vi "VelocityCommand.vi"(5 "intervalo":dbl=0.016, 7 "estimatives":T1, 8 "Velocities Y":dbl[](array[numeric]), 9 "Time Y":dbl[](array[numeric]), 10 "Velocities X":dbl[](array[numeric]), 11 "Time X":dbl[](array[numeric])) -> (1 "Vy":dbl, 2 "Vx":dbl)   [LabVIEW 2018]
panel:
  out "Velocity Profile Y":cluster{dbl[], dbl[]}[](graph)
  out "Velocity Profile X":cluster{dbl[], dbl[]}[](graph)
  in  "est_vx":dbl
  in  "est_vy":dbl
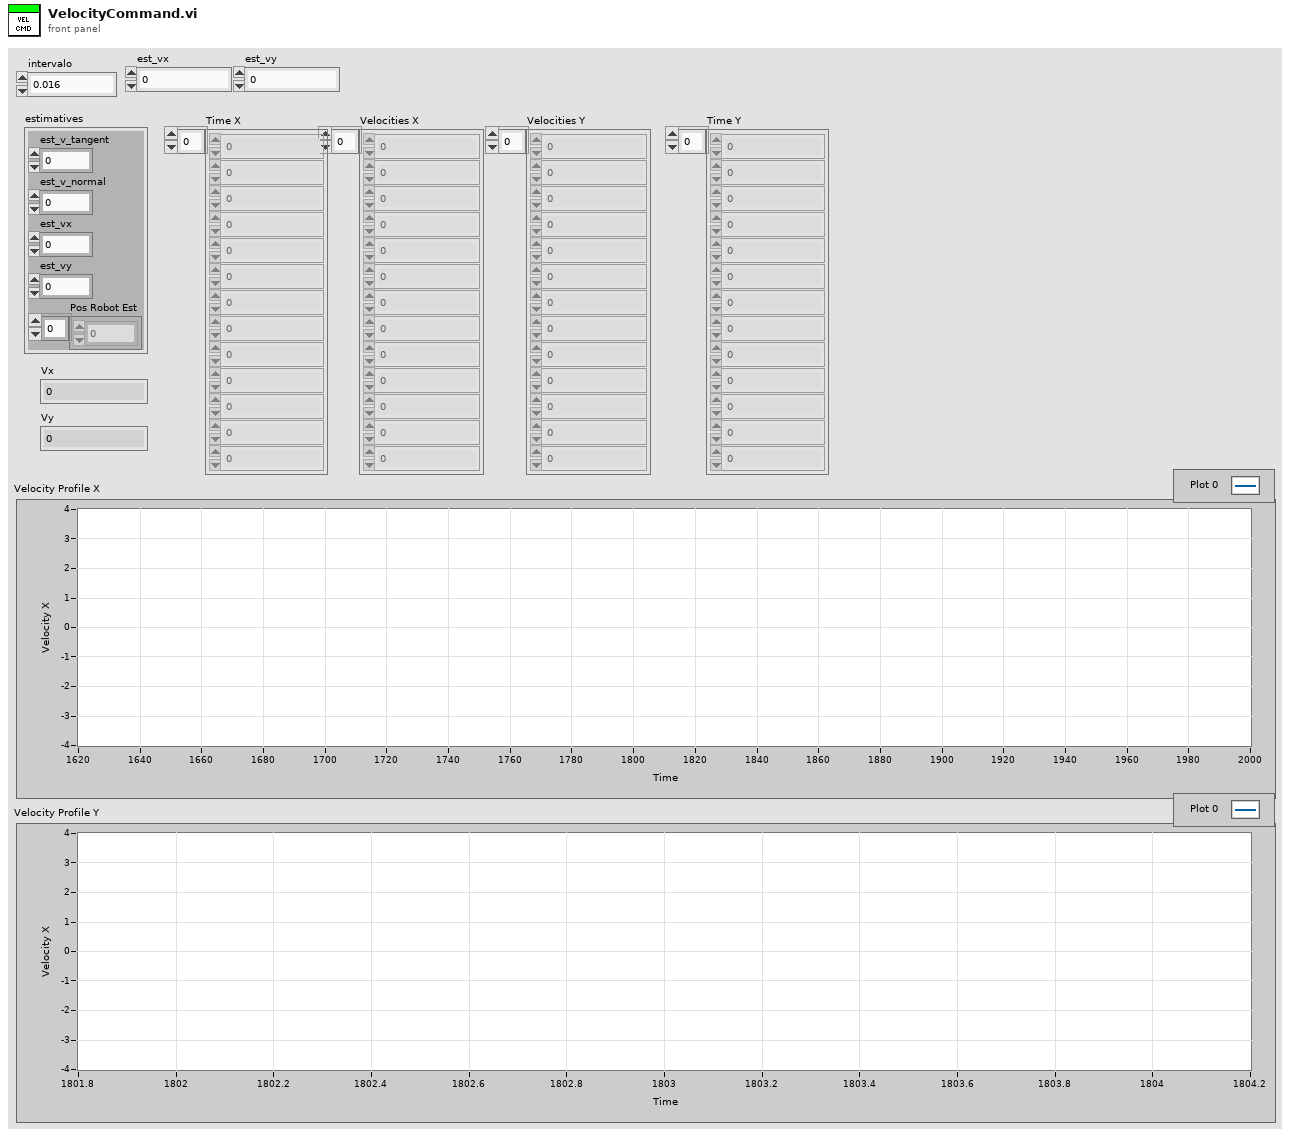
[diagram p1: front panel]
types:
  T1 = cluster{"est_v_tangent":dbl, "est_v_normal":dbl, "est_vx":dbl, "est_vy":dbl, "Pos Robot Est":dbl[]}
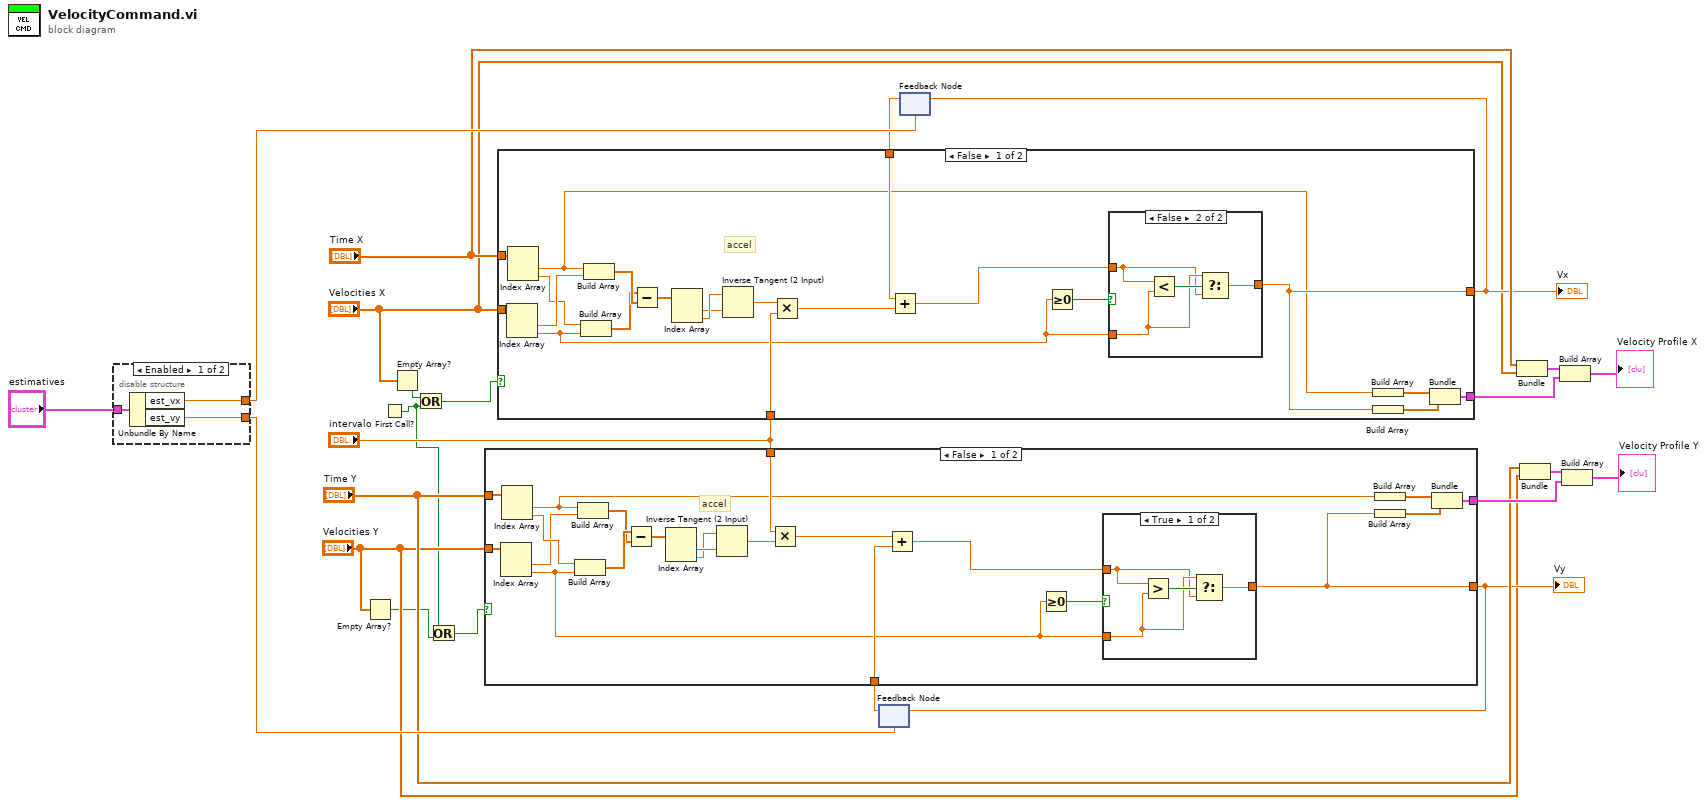
[diagram p0: block diagram]
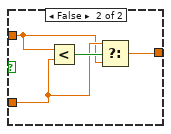
[diagram p2: hidden frame]
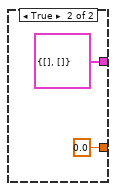
[diagram p3: hidden frame]
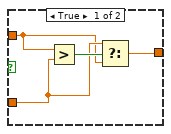
[diagram p4: hidden frame]
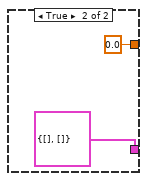
[diagram p5: hidden frame]
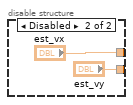
[diagram p6: hidden frame]
diagram:
  n1 = disable-structure shown="Enabled" {
    disable-tunnel: "estimatives" -> [w26 _]
    disable-tunnel: [w25 "est_vx"] -> w22
    disable-tunnel: [w24 "est_vy"] -> w20
    frame Enabled {
      n2 = Unbundle By Name(w26) -> ("est_vx"=w25:dbl, "est_vy"=w24:dbl)
    }
    frame Disabled {
    }
  }
  n3 = Empty Array?(array="Velocities Y") -> (empty?=w3:bool)
  n4 = First Call?() -> (First Call?: T/F=w2:bool)
  n5 = Empty Array?(array="Velocities X") -> (empty?=w5:bool)
  n6 = Or(x=w5, y=w2) -> (x .or. y?=w4:bool)
  n7 = Or(x=w2, y=w3) -> (x .or. y?=w1:bool)
  n8 = feedback #1(w20) -> (w8:dbl)
  n9 = case shown="False" w1 {
    tunnel: "intervalo" -> [w49 _]
    tunnel: [w48 cluster{dbl[], dbl[]} {[], []}] -> w15
    tunnel: "Velocities Y" -> [w47 _]
    tunnel: "Time Y" -> [w46 _]
    tunnel: w8 -> [w45 _]
    tunnel: [w44 0.0 ("v3")] -> w7
    frame False {
      # "accel"
      n10 = Index Array(array=w47) -> (element #1=w37:dbl, element #2=w32:dbl)  [unwired: 2 in]
      n11 = Index Array(array=w46) -> (element #1=w29:dbl, element #2=w38:dbl)  [unwired: 2 in]
      n12 = Build Array(w38, w32) -> (w40:dbl[])
      n13 = Build Array(w29, w37) -> (w39:dbl[])
      n14 = Subtract(x=w40, y=w39) -> (x-y=w41:dbl[])
      n15 = Index Array(array=w41) -> (element #1=w43:dbl, element #2=w42:dbl)  [unwired: 2 in]
      n16 = Inverse Tangent (2 Input)(1:w43, 2:w42) -> (0:w36:dbl)
      n17 = Multiply(x=w49, y=w36) -> (x*y=w35:dbl)
      n18 = Add(x=w35, y=w45) -> (x+y=w33:dbl)
      n19 = Greater Or Equal To 0?(x=w32) -> (x >= 0?=w34:bool)
      n20 = case shown="True" w34 {
        tunnel: w33 -> [w51 w55]
        tunnel: w32 -> [w52 w56]
        tunnel: [w50 w54] -> w44
        frame True {
          n21 = Greater?(x=w51, y=w52) -> (0:w53:bool)
          n22 = Select(t=w52, s=w53, f=w51) -> (s? t:f=w50:dbl)
        }
        frame False {
          n23 = Less?(x=w55, y=w56) -> (x < y?=w57:bool)
          n24 = Select(t=w56, s=w57, f=w55) -> (s? t:f=w54:dbl)
        }
      }
      n25 = Build Array(w29) -> (w31:dbl[])
      n26 = Build Array(w44) -> (w30:dbl[])
      n27 = Bundle(w31, w30) -> (w48:cluster{dbl[], dbl[]})  [unwired: 1 in]
    }
    frame True {
    }
  }
  "Vy" <- w7
  n28 = feedback-in #1(w7) -> ()
  n29 = feedback #2(w22) -> (w11:dbl)
  n30 = case shown="False" w4 {
    tunnel: "intervalo" -> [w80 _]
    tunnel: [w79 cluster{dbl[], dbl[]} {[], []} ("Cluster")] -> w17
    tunnel: "Time X" -> [w78 _]
    tunnel: w11 -> [w77 _]
    tunnel: [w76 0.0 ("v3")] -> w10
    tunnel: "Velocities X" -> [w75 _]
    frame False {
      # "accel"
      n31 = Index Array(array=w75) -> (element #1=w74:dbl, element #2=w63:dbl)  [unwired: 2 in]
      n32 = Index Array(array=w78) -> (element #1=w60:dbl, element #2=w73:dbl)  [unwired: 2 in]
      n33 = Build Array(w73, w63) -> (w71:dbl[])
      n34 = Build Array(w60, w74) -> (w72:dbl[])
      n35 = Subtract(x=w71, y=w72) -> (x-y=w70:dbl[])
      n36 = Index Array(array=w70) -> (element #1=w68:dbl, element #2=w69:dbl)  [unwired: 2 in]
      n37 = Inverse Tangent (2 Input)(1:w68, 2:w69) -> (0:w67:dbl)
      n38 = Multiply(x=w67, y=w80) -> (x*y=w66:dbl)
      n39 = Add(x=w77, y=w66) -> (x+y=w64:dbl)
      n40 = Greater Or Equal To 0?(x=w63) -> (x >= 0?=w65:bool)
      n41 = case shown="False" w65 {
        tunnel: w64 -> [w82 w86]
        tunnel: w63 -> [w83 w87]
        tunnel: [w81 w85] -> w76
        frame True {
          n42 = Greater?(x=w82, y=w83) -> (0:w84:bool)
          n43 = Select(t=w83, s=w84, f=w82) -> (s? t:f=w81:dbl)
        }
        frame False {
          n44 = Less?(x=w86, y=w87) -> (x < y?=w88:bool)
          n45 = Select(t=w87, s=w88, f=w86) -> (s? t:f=w85:dbl)
        }
      }
      n46 = Build Array(w60) -> (w61:dbl[])
      n47 = Build Array(w76) -> (w62:dbl[])
      n48 = Bundle(w61, w62) -> (w79:cluster{dbl[], dbl[]})  [unwired: 1 in]
    }
    frame True {
    }
  }
  "Vx" <- w10
  n49 = feedback-in #2(w10) -> ()
  n50 = Bundle("Time X"="Time X", "Velocities X"="Velocities X") -> (w19:cluster{"Time X":dbl[], "Velocities X":dbl[]})  [unwired: 1 in]
  n51 = Bundle("Time Y"="Time Y", "Velocities Y"="Velocities Y") -> (w13:cluster{"Time Y":dbl[], "Velocities Y":dbl[]})  [unwired: 1 in]
  n52 = Build Array(w19, w17) -> (→"Velocity Profile X":cluster{"Time X":dbl[], "Velocities X":dbl[]}[])
  n53 = Build Array(w13, w15) -> (→"Velocity Profile Y":cluster{"Time Y":dbl[], "Velocities Y":dbl[]}[])
